vi "Enable Output.vi"(8 "error in (no error)":errorcluster, 9 "Enable Type N Output (T: Enable)":bool=TRUE, 10 "Enable Low Frequency Output (T: Enable)":bool=TRUE, 11 "VISA resource name":refnum<visa-resource-name>) -> (0 "error out":errorcluster, 3 "VISA resource name out":refnum<visa-resource-name>)   [LabVIEW 2015, in "Stanford Research SG39x Series.lvlib"]
doc: "Enables or disables the output connectors."
uses:
  Stanford Research SG39x Series.lvlib
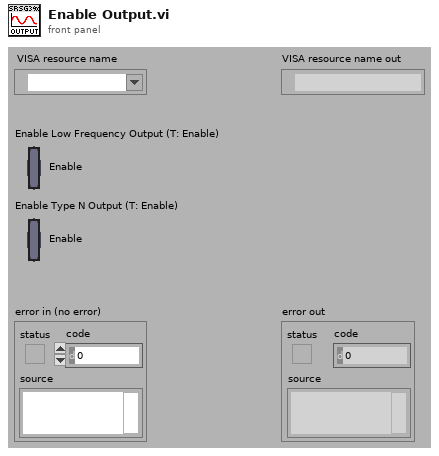
[diagram p1: front panel]
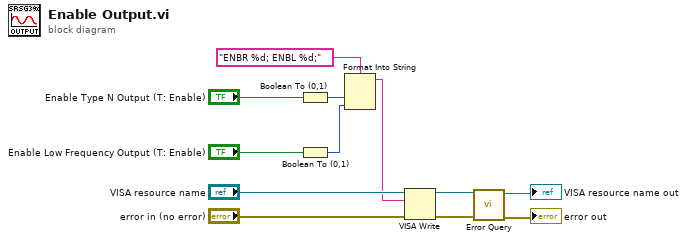
[diagram p0: block diagram]
diagram:
  n1 = Boolean To (0,1)(Boolean="Enable Type N Output (T: Enable)") -> (0, 1=w6:i16)
  n2 = Boolean To (0,1)(Boolean="Enable Low Frequency Output (T: Enable)") -> (0, 1=w2:i16)
  n3 = Format Into String(format string="ENBR %d; ENBL %d;" ("true string"), w6, w2) -> (resulting string=w1:string)  [unwired: 2 in, 1 out]
  n4 = VISA Write(VISA resource name="VISA resource name", write buffer=w1, error in (no error)="error in (no error)") -> (VISA resource name out=w10:refnum<visa-resource-name>, error out=w9:errorcluster)  [unwired: 1 out]
  n5 = call "Error Query.vi"("error in (no error)"=w9, "VISA resource name"=w10) -> ("error out"=→"error out":errorcluster, "VISA resource name out"=→"VISA resource name out":refnum<visa-resource-name>)  [unwired: 6 in, 2 out]
